vi "RandomUint8.vi"() -> (3 "RandomUint8":u8)   [LabVIEW 2009]
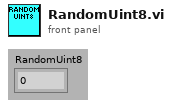
[diagram p1: front panel]
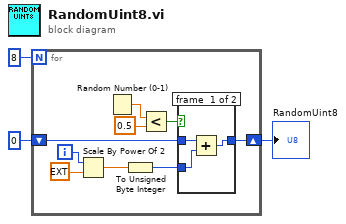
[diagram p0: block diagram]
diagram:
  n1 = for {
    N: 8 -> [_]
    shift-right: [w6] -> w1
    shift-left: u8 0 ("XORByte") -> [w8]
    i -> [w12]
    n2 = Scale By Power Of 2(n=w12, x=ext 1.0) -> (x*2^n=w5:ext)
    n3 = Random Number (0-1)() -> (number: 0 to 1=w9:dbl)
    n4 = To Unsigned Byte Integer(number=w5) -> (unsigned 8bit integer=w4:u8)
    n5 = Less?(x=w9, y=0.5) -> (x < y?=w7:bool)
    n6 = case shown="False" w7 {
      tunnel: w8 -> [w14 w16]
      tunnel: [w13 w16] -> w6
      tunnel: w4 -> [w15 _]
      frame #0 {
        n7 = Add(x=w14, y=w15) -> (x+y=w13:u8)
      }
      frame #1 {
      }
    }
  }
  "RandomUint8" <- w1
